vi "templates new template.vi"(6 "user":string, 7 "POST Parameters":T1, 8 "error in":errorcluster, 9 "Keys in":T1, 10 "template STYLE":string, 11 "Connection Refnum":T2) -> (0 "error out":errorcluster, 1 "HTM Keys out":T1, 2 "sEditor":string, 3 "Connection Refnum 2":T2)   [LabVIEW 2011]
uses:
  ITK EXT/utils/keyedarr.llb/Keyed Array.ctl
  Summitek EXT/ODBC/SQL Controls/Connection Refnum.ctl
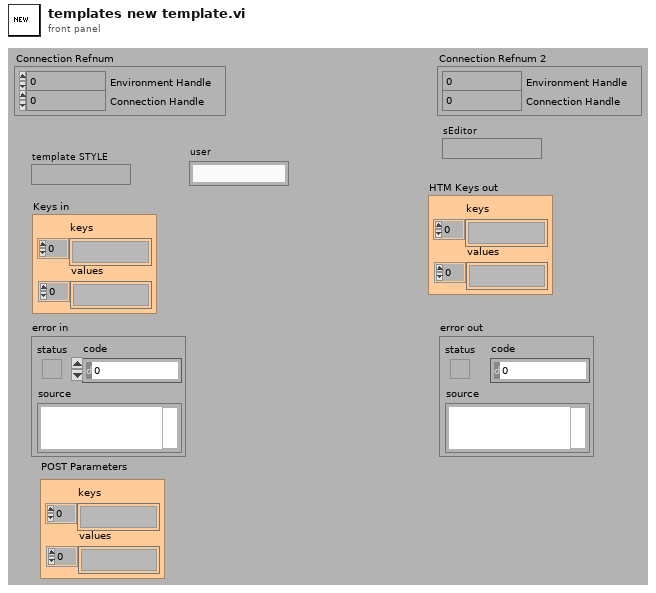
[diagram p1: front panel]
types:
  T1 = typedef "Keyed Array.ctl" = cluster{"keys":string[], "values":string[]}
  T2 = typedef "Connection Refnum.ctl" = cluster{"Environment Handle":i32, "Connection Handle":i32}
  T3 = typedef "Template Record.ctl" = cluster{"ixTemplate":i32, "sxTemplateId":string, "sDescription":string, "sCreator":string, "tCreationDate":timestamp, "sModifier":string, "tModifiedDate":timestamp, "sType":string, "sStyle":string, "sFormat":string, "dWidth":dbl, "dHeight":dbl, "sFilename":string, "sScript":string, "sLayout":string, "sEditor":string, "sStyleProcess":string}
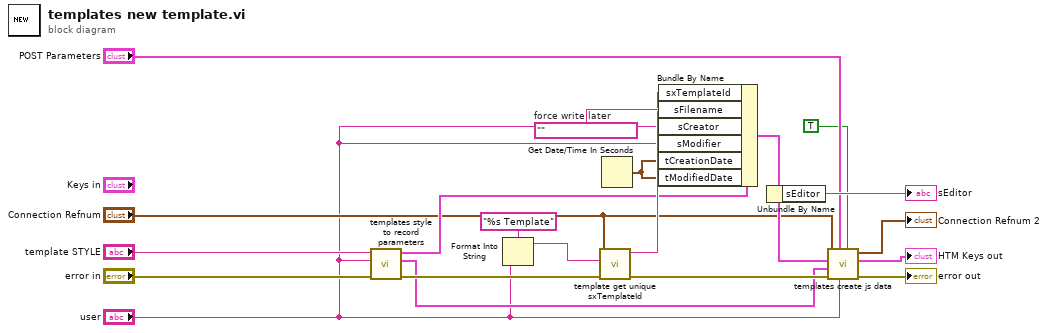
[diagram p0: block diagram]
diagram:
  w13 = ""  # force write later
  n1 = call "templates style to record parameters.vi"("error in (no error)"="error in", "user"="user", "template style"="template STYLE") -> ("error out"=w11:errorcluster, "Parameters"=w6:T1, "Template Record"=w10:T3)  [unwired: 6 out]
  n2 = Format Into String(format string="%s Template" ("template STYLE"), "user") -> (resulting string=w4:string)  [unwired: 2 in, 1 out]
  n3 = call "template get unique sxTemplateId.vi"("error in"=w11, "sxTemplateId proposed"=w4, "Connection Refnum"="Connection Refnum") -> ("error out"=w8:errorcluster, "sxTemplateId"=w12:string)  [unwired: 7 out]
  n4 = Get Date/Time In Seconds() -> (seconds since 1Jan1904=w1:timestamp)
  n5 = Bundle By Name(cluster=w10, "sxTemplateId"=w12, "sFilename"=w13, "sCreator"="user", "sModifier"="user", "tCreationDate"=w1, "tModifiedDate"=w1) -> (w9:T3)
  n6 = Unbundle By Name(w9) -> ("sEditor"=→"sEditor":string)
  n7 = call "templates create js data.vi"("Changes?"=TRUE, "sxUsername"="user", "POST Parameters"="POST Parameters", "error in (no error)"=w8, "template Parameters"=w6, "Template Record"=w9, "Connection Refnum"="Connection Refnum") -> ("error out"=→"error out":errorcluster, "HTM Keys"=→"HTM Keys out":T1, "Connection Refnum"=→"Connection Refnum 2":T2)  [unwired: 2 out]
